vi "defaultConfiguration.vi"(8 "error in (no error)":errorcluster, 11 "Camera in":refnum<class "Camera.lvclass">) -> (0 "error out":errorcluster, 3 "Camera out":refnum<class "Camera.lvclass">)   [LabVIEW 2020, in "Camera.lvclass"]
doc: "Sets the camera to it’s default configuration. This function is also called during initialization inside\ninit.vi and init_ex.vi."
uses:
  Camera.lvclass
  Camera.lvclass/Camera.ctl
  RecordingControl.lvlib
  GeneralCameraControl.lvlib
  ImageInformation.lvlib
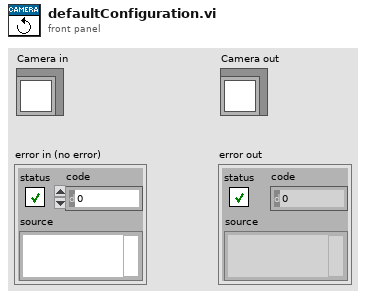
[diagram p1: front panel]
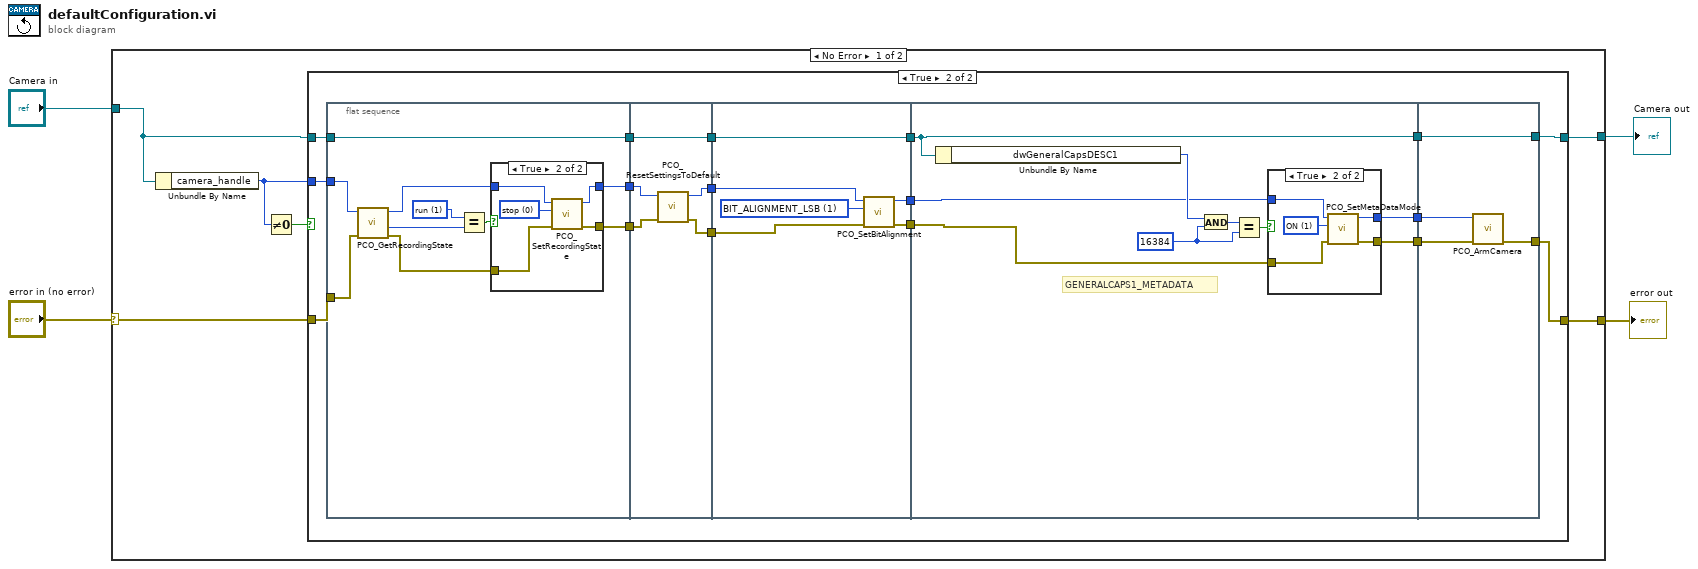
[diagram p0: block diagram]
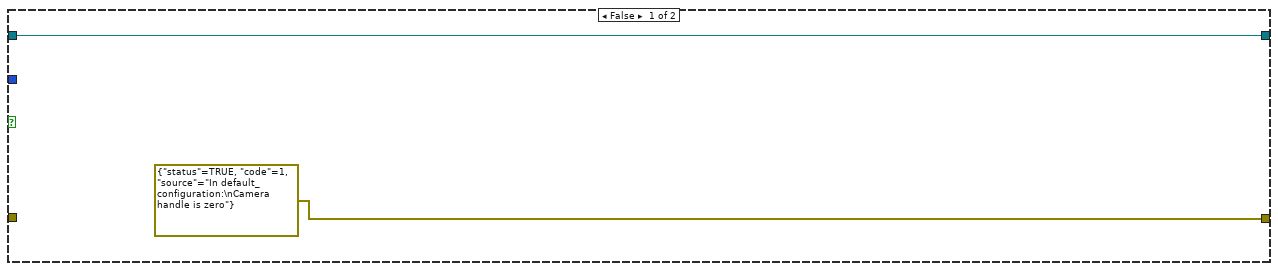
[diagram p2: hidden frame]
diagram:
  n1 = case shown="No Error" "error in (no error)" {
    selector: "error in (no error)" -> [w8 w79]
    tunnel: [w7 w79] -> w3
    tunnel: [w5 w78] -> w1
    tunnel: "Camera in" -> [w6 w78]
    frame No Error {
      n2 = Unbundle By Name(w6) -> ("camera_handle"=w9:u64)
      n3 = Not Equal To 0?(x=w9) -> (x != 0?=w10:bool)
      n4 = case shown="True" w10 {
        tunnel: [errorcluster {"status"=TRUE, "code"=1, "source"="In default_configuration:\nCamera handle is zero"} ("error constant") w13] -> w7
        tunnel: w9 -> [_ w28]
        tunnel: w8 -> [_ w29]
        tunnel: w6 -> [w11 w20]
        tunnel: [w11 w14] -> w5
        frame False {
        }
        frame True {
          n5 = flat-sequence {
            tunnel: w29 -> [w39]
            tunnel: w28 -> [w38]
            tunnel: [w33] -> w27
            tunnel: [w31] -> w26
            tunnel: [w30] -> w21
            tunnel: w20 -> [w30]
            tunnel: w27 -> [w51]
            tunnel: w26 -> [w50]
            tunnel: [w49] -> w25
            tunnel: [w48] -> w24
            tunnel: w21 -> [w47]
            tunnel: [w47] -> w18
            tunnel: w25 -> [w57]
            tunnel: w24 -> [w56]
            tunnel: [w55] -> w23
            tunnel: [w54] -> w22
            tunnel: [w53] -> w19
            tunnel: w18 -> [w53]
            tunnel: w23 -> [w61]
            tunnel: w22 -> [w62]
            tunnel: w19 -> [w58]
            tunnel: [w60] -> w17
            tunnel: [w59] -> w16
            tunnel: [w58] -> w15
            tunnel: [w77] -> w13
            tunnel: w17 -> [w76]
            tunnel: w16 -> [w75]
            tunnel: [w74] -> w14
            tunnel: w15 -> [w74]
            frame #0 {
              w36 = u16 1 items=["stop", "run"] ("wRecState")
              n6 = call "PCO_GetRecordingState.vi"("error in (no error)"=w39, "ph"=w38) -> ("error out"=w34:errorcluster, "wRecState"=w37:u16, "ph out"=w32:u64)  [unwired: 6 in, 1 out]
              n7 = Equal?(x=w36, y=w37) -> (x = y?=w35:bool)
              n8 = case shown="True" w35 {
                tunnel: w34 -> [w41 w45]
                tunnel: [w41 w44] -> w33
                tunnel: w32 -> [w40 w43]
                tunnel: [w40 w42] -> w31
                frame False {
                }
                frame True {
                  w46 = u16 0 items=["stop", "run"] ("wRecState")
                  n9 = call "PCO_SetRecordingState.vi"("error in (no error)"=w45, "wRecState"=w46, "ph"=w43) -> ("error out"=w44:errorcluster, "ph out"=w42:u64)  [unwired: 6 in, 1 out]
                }
              }
            }
            frame #1 {
              n10 = call "PCO_ResetSettingsToDefault.vi"("error in (no error)"=w51, "ph"=w50) -> ("error out"=w49:errorcluster, "ph out"=w48:u64)  [unwired: 7 in, 1 out]
            }
            frame #2 {
              w52 = u16 1 items=["BIT_ALIGNMENT_MSB", "BIT_ALIGNMENT_LSB"] ("wBitAlignment")
              n11 = call "PCO_SetBitAlignment.vi"("error in (no error)"=w57, "wBitAlignment"=w52, "ph"=w56) -> ("error out"=w54:errorcluster, "ph out"=w55:u64)  [unwired: 6 in, 1 out]
            }
            frame #3 {
              w65 = u32 16384 ("y")
              # "GENERALCAPS1_METADATA"
              n12 = Unbundle By Name(w58) -> ("dwGeneralCapsDESC1"=w63:u32)
              n13 = And(x=w63, y=w65) -> (x .and. y?=w66:u32)
              n14 = Equal?(x=w66, y=w65) -> (x = y?=w64:bool)
              n15 = case shown="True" w64 {
                tunnel: w62 -> [w67 w71]
                tunnel: w61 -> [w68 w72]
                tunnel: [w67 w70] -> w59
                tunnel: [w68 w69] -> w60
                frame False {
                }
                frame True {
                  w73 = u16 1 items=["OFF", "ON"] ("wMetaDataMode")
                  n16 = call "PCO_SetMetaDataMode.vi"("error in (no error)"=w71, "wMetaDataMode"=w73, "ph"=w72) -> ("error out"=w70:errorcluster, "ph out"=w69:u64)  [unwired: 4 in, 3 out]
                }
              }
            }
            frame #4 {
              n17 = call "PCO_ArmCamera.vi"("error in (no error)"=w75, "ph"=w76) -> ("error out"=w77:errorcluster)  [unwired: 7 in, 2 out]
            }
          }
        }
      }
    }
    frame Error {
    }
  }
  "error out" <- w3
  "Camera out" <- w1
